vi "Validate_RegDests.vi"(8 "error in (no error)":errorcluster, 11 "IB_MSI in":refnum<class "IB_MSI.lvclass">) -> (0 "error out":errorcluster, 3 "IB_MSI out":refnum<class "IB_MSI.lvclass">)   [LabVIEW 2020, in "IB_MSI.lvclass"]
uses:
  <vilib>/AppBuilder/IB_Classes/MSI/IB_MSI.lvclass
  <vilib>/AppBuilder/IB_Classes/MSI/IB_MSI.lvclass/IB_MSI.ctl
  <vilib>/AppBuilder/IB_Classes/RegGroup/IB_RegGroup.lvclass
  <vilib>/AppBuilder/IB_Classes/RegDest/IB_RegDest.lvclass
  e:/builds/penguin/labview/branches/2020/dev/dist/vi.lib/AppBuilder/IB_Classes/Installer/Installer.lvclass
  e:/builds/penguin/labview/branches/2020/dev/dist/vi.lib/AppBuilder/IB_Classes/MSI/IB_MSI.lvclass
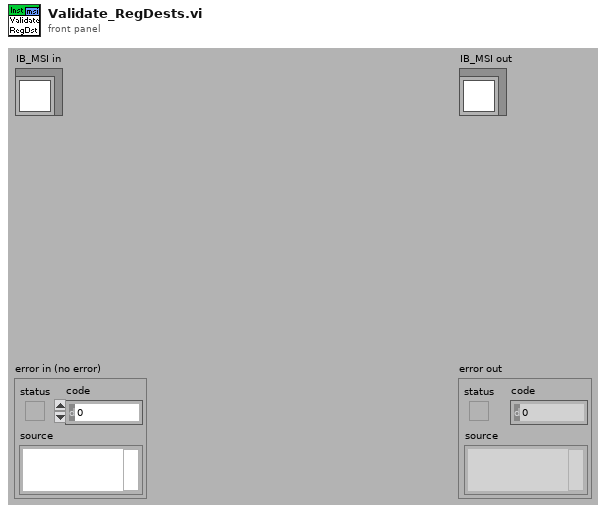
[diagram p1: front panel]
types:
  T1 = typedef "IB_RegDest.ctl" = cluster{"parentTag":string, "dirTag":string, "dirName":string, "unlock":bool, "path":string, "regData":refnum<class "IB_RegData.lvclass">[]}
  T2 = typedef "IB_RegGroup.ctl" = cluster{"RegData":refnum<class "IB_RegData.lvclass">[], "dirTag":string}
  T3 = cluster{"result string":string, "Class out":refnum<class "IB_RegDest.lvclass">}
  T4 = cluster{"result string":string, "Class out":refnum<class "IB_RegDest.lvclass">}[]
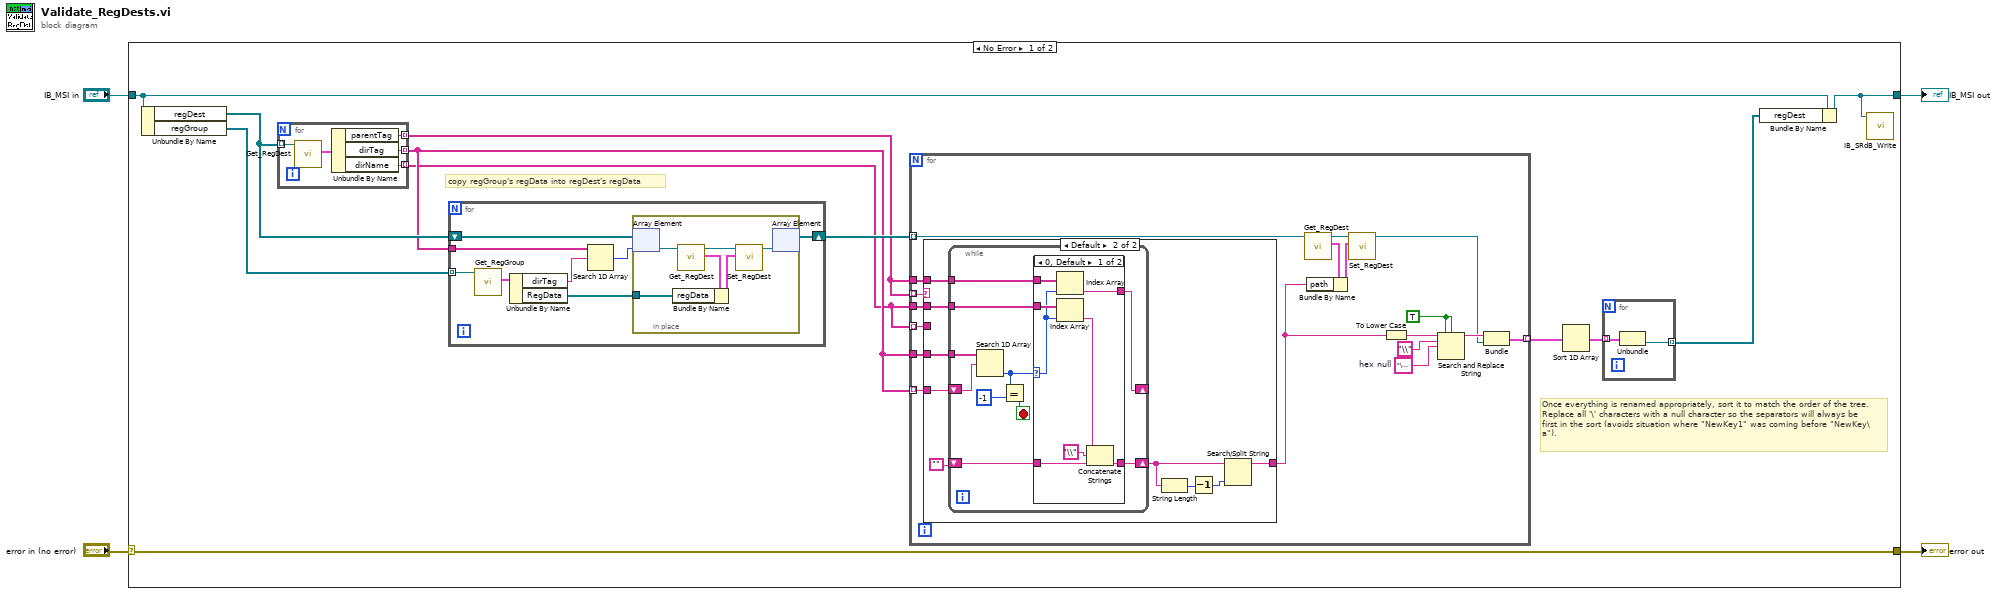
[diagram p0: block diagram]
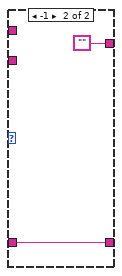
[diagram p3: hidden frame]
diagram:
  n1 = case shown="No Error" "error in (no error)" {
    selector: "error in (no error)" -> [w16 w87]
    tunnel: [w16 w87] -> w3
    tunnel: [w5 w86] -> w1
    tunnel: "IB_MSI in" -> [w13 w86]
    frame No Error {
      # "Once everything is renamed appropriately, sort it to match the order of the tree.  Replace all '\\' characters with a null character so the separators will always be first in the sort (avoids situation where \"NewKey1\" was coming before \"NewKey\\a\")."
      # "copy regGroup's regData into regDest's regData"
      n2 = Unbundle By Name(w13) -> ("regDest"=w14:refnum<class "IB_RegDest.lvclass">[], "regGroup"=w15:refnum<class "IB_RegGroup.lvclass">[])
      n3 = for {
        tunnel: w14 -> [w71] mode=indexing
        tunnel: [w69] -> w11 mode=indexing
        tunnel: [w68] -> w9 mode=indexing
        tunnel: [w67] -> w10 mode=indexing
        n4 = call <vilib>:"Get_RegDest.vi"("Class in"=w71) -> ("data"=w70:T1)  [unwired: 1 in, 9 out]
        n5 = Unbundle By Name(w70) -> ("parentTag"=w67:string, "dirTag"=w69:string, "dirName"=w68:string)
      }
      n6 = for {
        tunnel: w15 -> [w79] mode=indexing
        tunnel: w11 -> [w77]
        shift-right: [w72] -> w12
        shift-left: w14 -> [w74]
        n7 = call <vilib>:"Get_RegGroup.vi"("IB_RegGroup in"=w79) -> ("data"=w78:T2)  [unwired: 1 in, 9 out]
        n8 = Unbundle By Name(w78) -> ("dirTag"=w76:string, "RegData"=w75:refnum<class "IB_RegData.lvclass">[])
        n9 = Search 1D Array(1D array=w77, element=w76) -> (index of element=w73:i32)  [unwired: 1 out]
        n10 = in-place {
          in-place-border: w75 -> [w82]
          n11 = in-place-array #1(w74, w73) -> (w80:refnum<class "IB_RegDest.lvclass">)
          n12 = call <vilib>:"Get_RegDest.vi"("Class in"=w80) -> ("data"=w84:T1, "Class out"=w85:refnum<class "IB_RegDest.lvclass">)  [unwired: 1 in, 8 out]
          n13 = Bundle By Name(cluster=w84, "regData"=w82) -> (w83:T1)
          n14 = call <vilib>:"Set_RegDest.vi"("data"=w83, "Class in"=w85) -> ("Class out"=w81:refnum<class "IB_RegDest.lvclass">)  [unwired: 1 in, 8 out]
          n15 = in-place-array #1(w81) -> (w72:refnum<class "IB_RegDest.lvclass">[])  [unwired: 1 out]
        }
      }
      n16 = for {
        tunnel: w10 -> [w36]
        tunnel: w11 -> [w35]
        tunnel: w9 -> [w34]
        tunnel: w11 -> [w33] mode=indexing
        tunnel: w12 -> [w29] mode=indexing
        tunnel: w10 -> [w28] mode=indexing
        tunnel: w9 -> [w27] mode=indexing
        tunnel: [w19] -> w8 mode=indexing
        w25 = "\u0000"  # hex null
        w23 = TRUE ("replace all? (F)")
        n17 = case shown="Default" w28 {
          tunnel: w36 -> [_ w45]
          tunnel: w35 -> [_ w44]
          tunnel: w34 -> [_ w43]
          tunnel: w33 -> [_ w42]
          tunnel: [w37 w38] -> w20
          tunnel: w27 -> [w37 _]
          frame "" {
            # "If it's root level, dirName is path"
          }
          frame Default {
            n18 = while {
              tunnel: w45 -> [w54]
              tunnel: w43 -> [w53]
              shift-right: [w47] -> w39
              shift-left: "" -> [w48]
              shift-right: [w52] -> _
              shift-left: w42 -> [w56]
              tunnel: w44 -> [w55]
              stop <- w51 stop-if-true
              n19 = Search 1D Array(1D array=w55, element=w56) -> (index of element=w50:i32)  [unwired: 1 out]
              n20 = Equal?(x=w50, y=-1) -> (x = y?=w51:bool)
              n21 = case shown="0, Default" w50 {
                selector: w50 -> [w62 _]
                tunnel: w54 -> [w63 _]
                tunnel: w53 -> [w64 _]
                tunnel: [w61 ""] -> w52
                tunnel: w48 -> [w58 w66]
                tunnel: [w57 w66] -> w47
                frame 0, Default {
                  n22 = Index Array(array=w63, index=w62) -> (element=w61:string)
                  n23 = Index Array(array=w64, index=w62) -> (element=w60:string)
                  n24 = Concatenate Strings(w60, "\\" ("string"), w58) -> (w57:string)
                }
                frame -1 {
                }
              }
            }
            n25 = String Length(string=w39) -> (length=w41:i32)
            n26 = Decrement(x=w41) -> (x-1=w40:i32)
            n27 = Search/Split String(string=w39, offset (0)=w40) -> (substring before match=w38:string)  [unwired: 3 out]
          }
        }
        n28 = call <vilib>:"Get_RegDest.vi"("Class in"=w29) -> ("data"=w31:T1, "Class out"=w30:refnum<class "IB_RegDest.lvclass">)  [unwired: 1 in, 8 out]
        n29 = Bundle By Name(cluster=w31, "path"=w20) -> (w32:T1)
        n30 = call <vilib>:"Set_RegDest.vi"("data"=w32, "Class in"=w30) -> ("Class out"=w21:refnum<class "IB_RegDest.lvclass">)  [unwired: 1 in, 8 out]
        n31 = To Lower Case(string=w20) -> (all lower case string=w26:string)
        n32 = Search and Replace String(replace all?=w23, case sensitive?=w23, input string=w26, search string="\\", replace string=w25) -> (result string=w22:string)  [unwired: 1 in, 5 out]
        n33 = Bundle("result string"=w22, "Class out"=w21) -> (w19:T3)  [unwired: 1 out]
      }
      n34 = Sort 1D Array(array=w8) -> (sorted array=w7:T4)
      n35 = for {
        tunnel: w7 -> [w18] mode=indexing
        tunnel: [w17] -> w6 mode=indexing
        n36 = Unbundle(w18) -> ("Class out"=w17:refnum<class "IB_RegDest.lvclass">)  [unwired: 1 out]
      }
      n37 = Bundle By Name(cluster=w13, "regDest"=w6) -> (w5:refnum<class "IB_MSI.lvclass">)
      n38 = call <resource>:"IB_SRdB_Write.vi"("installer"=w5) -> ()  [unwired: 1 in, 10 out]
    }
    frame Error {
    }
  }
  "error out" <- w3
  "IB_MSI out" <- w1
